vi "PID Get Profiled Setpoint.vi"(11 "Data Value Reference in":refnum<data-value>) -> (1 "Velocity":dbl, 2 "Position":dbl, 3 "Data Value Reference out":refnum<data-value>)   [LabVIEW 2019]
uses:
  Typedef/PID Controller State.ctl
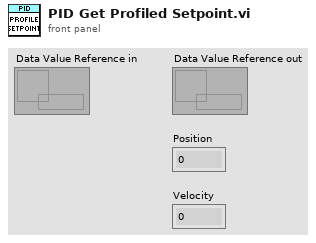
[diagram p1: front panel]
types:
  T1 = typedef "PID Controller State.ctl" = cluster{"PIDF Gains":cluster{"Kp":dbl, "Ki":dbl, "Kd":dbl, "Kf":dbl}, "Output Range":cluster{"output high":dbl, "output low":dbl}, "Profiled?":bool, "PID State":cluster{"iState":dbl, "dState":dbl, "Error [n-1]":dbl, "Output":dbl}, "Setpoint":dbl, "Profiled State":cluster{"Position":dbl, "Velocity":dbl}, "Profiled Contraints":cluster{"Max Velocity":dbl, "Max Acceleration":dbl}}
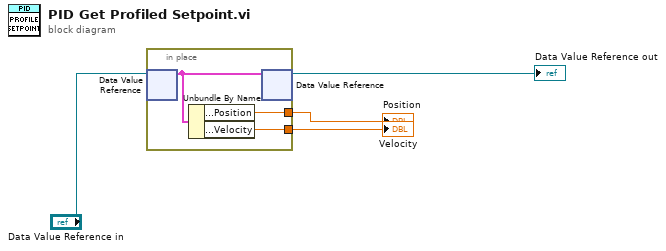
[diagram p0: block diagram]
diagram:
  n1 = in-place {
    in-place-border: [w7] -> w1
    in-place-border: [w6] -> w2
    n2 = in-place-dvr #1("Data Value Reference in") -> (w5:T1)  [unwired: 1 out]
    n3 = Unbundle By Name(w5) -> ("Profiled State.Position"=w7:dbl, "Profiled State.Velocity"=w6:dbl)
    n4 = in-place-dvr #1(w5) -> (→"Data Value Reference out":refnum<data-value>)  [unwired: 1 out]
  }
  "Velocity" <- w2
  "Position" <- w1
